vi "Cowl_Notifier_Begin.vi"   [LabVIEW 2020]
uses:
  Subsystems/Cowl/Cowl_Cluster.ctl
  Subsystems/Cowl/Cowl_States.ctl
  Globals/Cowl_Globals.vi
types:
  T1 = typedef "Cowl_Cluster.ctl" = cluster{"Control_State\n":T2, "Manual_Cowl_%Power":dbl}
  T2 = typedef "Cowl_States.ctl" = enum16{"Manual_%VBus", "GoToAngle"}
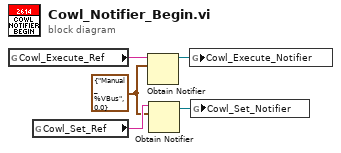
[diagram p0: block diagram]
diagram:
  w1 = T1 {"Control_State\n"=enum."Manual_%VBus", "Manual_Cowl_%Power"=0.0}
  n1 = global read "Cowl_Globals.vi" "Cowl_Execute_Ref"() -> (w2:string)
  n2 = global read "Cowl_Globals.vi" "Cowl_Set_Ref"() -> (w3:string)
  n3 = Obtain Notifier(name (unnamed)=w2, notification data type=w1) -> (notifier out=w4:refnum<notifier>)  [unwired: 2 in, 2 out]
  n4 = Obtain Notifier(name (unnamed)=w3, notification data type=w1) -> (notifier out=w5:refnum<notifier>)  [unwired: 2 in, 2 out]
  n5 = global write "Cowl_Globals.vi" "Cowl_Execute_Notifier"(w4) -> ()
  n6 = global write "Cowl_Globals.vi" "Cowl_Set_Notifier"(w5) -> ()
